vi "ObtainRequestEvents.vi"(8 "ErrorArray In":errorcluster[](array[cluster]), 10 "CreateNew (F)":bool) -> (0 "ErrorArray Out":errorcluster[](array[cluster]), 2 "clRequestEvents":T1)   [LabVIEW 2014, in "TestFramework.lvlib"]
uses:
  TestFramework.lvlib
  Protected/Requests/clRequestEvents.ctl
  Protected/clUserEventType.ctl
  <userlib>/NIST/NISTErrorLib/NISTErrorLib.lvlib
panel:
  # "If you want to add other Request Events, open this typedef, copy an existing event and rename it to your event name."
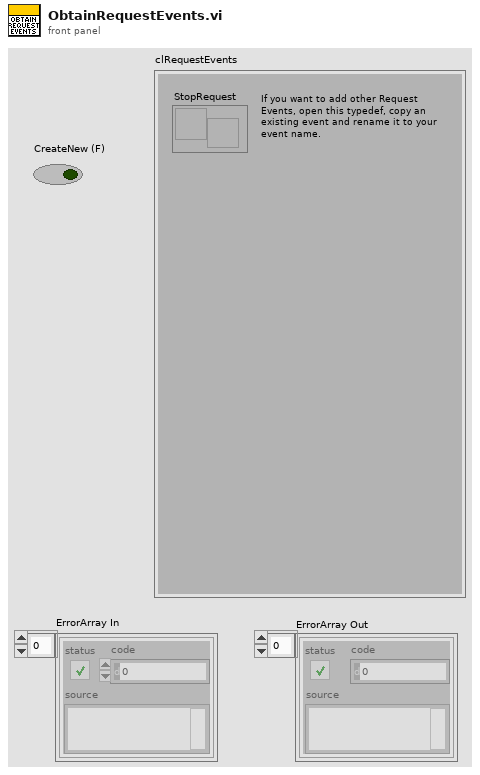
[diagram p1: front panel]
types:
  T1 = typedef "TestFramework.lvlib/clRequestEvents.ctl" = cluster{"StopRequest":refnum<user-event>}
  T2 = typedef "TestFramework.lvlib/clUserEventType.ctl" = cluster{"BusIndex":i8, "Data":variant}
  T3 = typedef "NISTFramework.lvlib/clRequestEvents.ctl" = cluster{"StopRequest":refnum<user-event>}
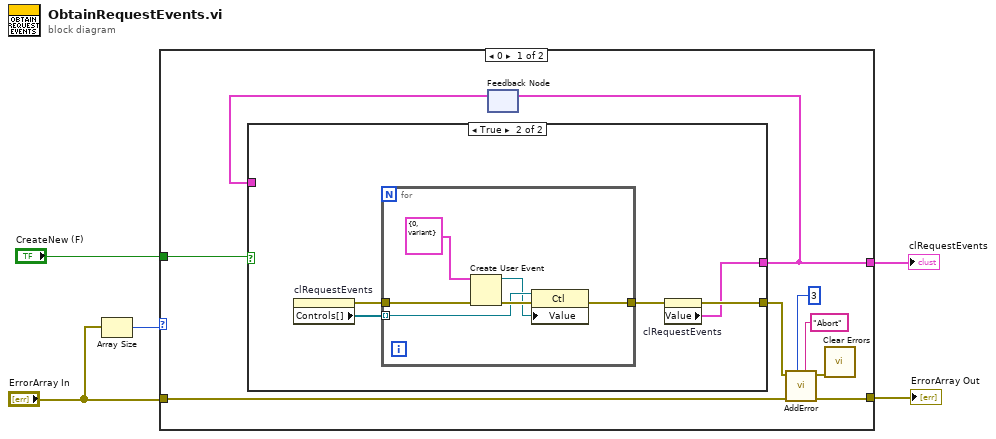
[diagram p0: block diagram]
diagram:
  n1 = Array Size(array="ErrorArray In") -> (size(s)=w3:i32)
  n2 = case shown="0" w3 {
    tunnel: "CreateNew (F)" -> [w14 _]
    tunnel: [w13 _] -> w4
    tunnel: [w8 w27] -> w1
    tunnel: "ErrorArray In" -> [w7 w27]
    frame 0 {
      n3 = feedback #1() -> (w12:T3)  [unwired: 1 in]
      n4 = case shown="True" w14 {
        tunnel: [_ w17] -> w6
        tunnel: [w15 w16] -> w13
        tunnel: w12 -> [w15 _]
        frame False {
        }
        frame True {
          n5 = property on="clRequestEvents" class="Clust (strict)"() -> (error out=w20:errorcluster, "Controls[]"=w19:refnum<vi>[])  [unwired: 2 in, 1 out]
          n6 = for {
            tunnel: w20 -> [w25]
            tunnel: w19 -> [w23] mode=indexing
            tunnel: [w21] -> w18
            n7 = Create User Event(user event datatype=T2 {"BusIndex"=0, "Data"=variant} ("clEventType"), error in=w25) -> (user event=w22:refnum<user-event>, error out=w24:errorcluster)
            n8 = property class="Ctl"(reference=w23, error in=w24, "Value"=w22) -> (error out=w21:errorcluster)  [unwired: 1 out]
          }
          n9 = property on="clRequestEvents" class="Clust (strict)"(error in=w18) -> (error out=w17:errorcluster, "Value"=w16:T3)  [unwired: 1 in, 1 out]
        }
      }
      n10 = feedback-in #1(w13) -> ()
      n11 = call <userlib>:"AddError.vi"("Severity"="Abort" ("String"), "Priority"=u8 3, "ErrorArray"=w7, "error in (no error)"=w6) -> ("ErrorArray"=w8:errorcluster[], "error out"=w11:errorcluster)  [unwired: 6 in]
      n12 = call <vilib>:"Clear Errors.vi"("error in (no error)"=w11) -> ()  [unwired: 5 in, 2 out]
    }
    frame 1, Default {
    }
  }
  "clRequestEvents" <- w4
  "ErrorArray Out" <- w1
